vi "ATMonochromator_monitorCommand_changeWavelength.vi"(8 "error in (no error)":errorcluster, 11 "command_changeWavelength_Ctl":T1) -> (0 "error out":errorcluster, 2 "function return":i32, 3 "command_changeWavelength_Ctl out":T1)   [LabVIEW 2016, in "SALLV_ATMonochromator.lvlib"]
doc: "int ATMonochromator_shm_monitorCommand_changeWavelengthLV(ATMonochromator_command_changeWavelengthLV *command_changeWavelength_Ctl );"
uses:
  SALLV_ATMonochromator.lvlib
  DataTypes/command_changeWavelength.ctl
  SALLV_ATMonochromator.so
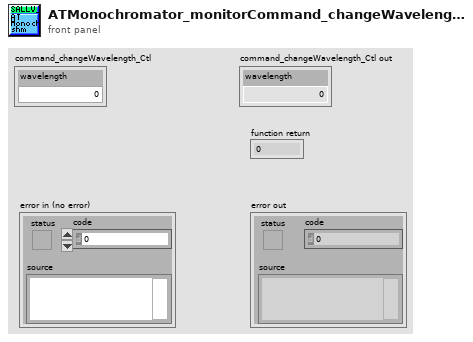
[diagram p1: front panel]
types:
  T1 = typedef "SALLV_ATMonochromator.lvlib/command_changeWavelength.ctl" = cluster{"wavelength":sgl}
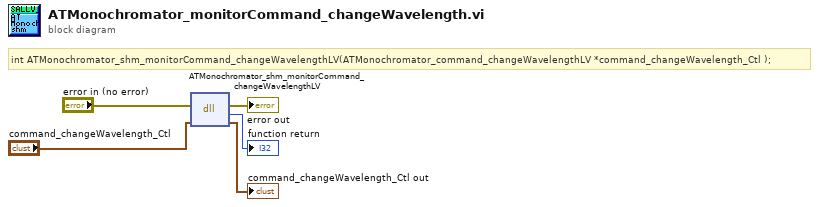
[diagram p0: block diagram]
diagram:
  # "int ATMonochromator_shm_monitorCommand_changeWavelengthLV(ATMonochromator_command_changeWavelengthLV *command_changeWavelength_Ctl );"
  n1 = dll-call lib="home/harini/tcs/SALLV_ATMonochromator/SALLV_ATMonochromator.*" fn="ATMonochromator_shm_monitorCommand_changeWavelengthLV"(error in="error in (no error)", "command_changeWavelength_Ctl"="command_changeWavelength_Ctl") -> (error out=→"error out":errorcluster, →"function return":i32, "command_changeWavelength_Ctl"=→"command_changeWavelength_Ctl out":T1)  [unwired: 2 in, 1 out]
